vi "io_write.vi"(6 "Block Logging (F)":bool, 8 "error in":errorcluster, 10 "write buffer":string, 11 "VISA resource name":refnum<visa-resource-name>) -> (0 "error out":errorcluster, 3 "VISA resource name out":refnum<visa-resource-name>)   [LabVIEW 2014, in "rszvl_rsidr_core.lvlib"]
uses:
  rszvl_rsidr_core.lvlib
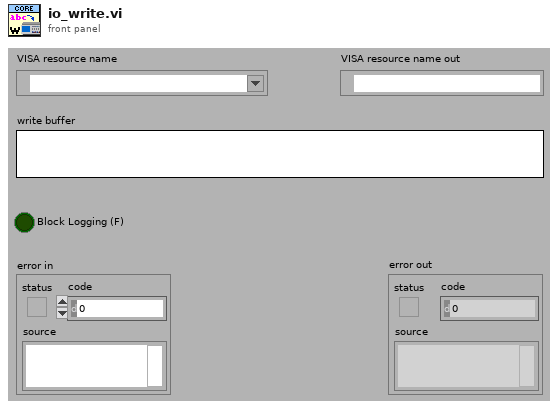
[diagram p1: front panel]
types:
  T1 = typedef "rszvl_rsidr_core.lvlib/type_Session_Data.ctl" = cluster{"Instr type":string, "Instr type for err. msg.":string, "Installed Options":string[], "OPC Timeout":i32, "Query Instrument Status":bool, "Check Range":bool, "Check Options":bool, "Add LF to Write":bool, "Simulate":bool, "Logging":bool, "Logging params":variant, "Interface Type":enum16{"Unknown", "GPIB", "VXI", "GPIB_VXI", "ASRL", "PXI", "TCPIP", "USB", "SOCKET"}, "Fast Sweep":i32, "AdditionalFlags":i32, "WaitBeforeWrite":i32, "WaitBeforeRead":i32, "BinDataChunkSize":i64}
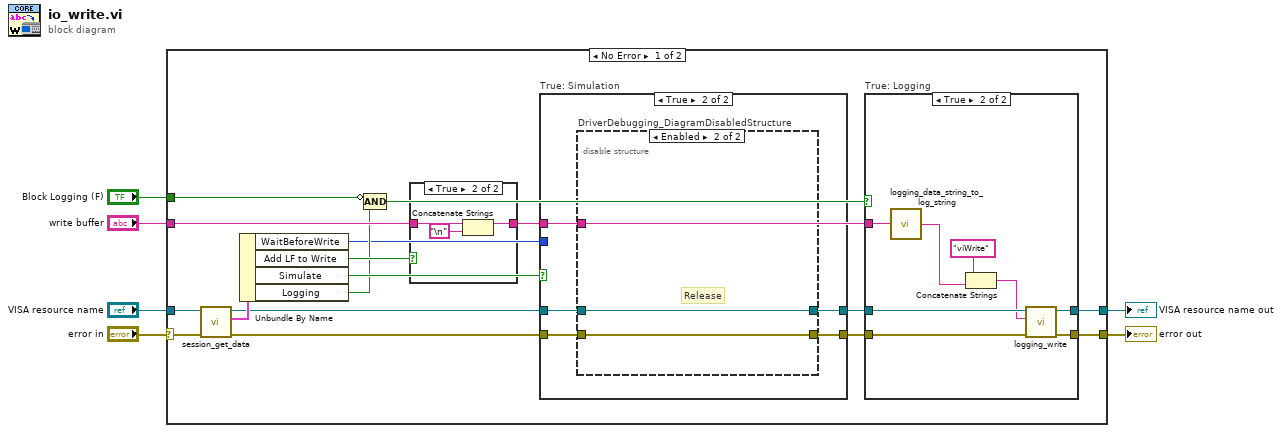
[diagram p0: block diagram]
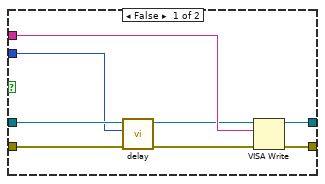
[diagram p3: hidden frame]
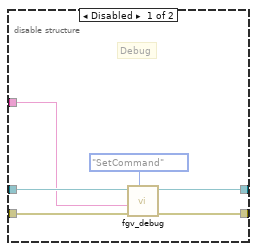
[diagram p4: hidden frame]
diagram:
  n1 = case shown="No Error" "error in" {
    selector: "error in" -> [w20 w60]
    tunnel: [w13 w59] -> w2
    tunnel: [w14 w60] -> w3
    tunnel: "write buffer" -> [w23 _]
    tunnel: "VISA resource name" -> [w19 w59]
    tunnel: "Block Logging (F)" -> [w7 _]
    frame No Error {
      n2 = call "session_get_data.vi"("error in"=w20, "VISA resource name"=w19) -> ("error out"=w18:errorcluster, "Session User Data out"=w21:T1, "VISA resource name out"=w10:refnum<visa-resource-name>)  [unwired: 7 in]
      n3 = Unbundle By Name(w21) -> ("WaitBeforeWrite"=w8:i32, "Add LF to Write"=w22:bool, "Simulate"=w17:bool, "Logging"=w16:bool)
      n4 = Compound Arithmetic op=AND(invert w7, w16) -> (w12:bool)
      n5 = case shown="True" w22 {
        tunnel: w23 -> [w55 w57]
        tunnel: [w55 w58] -> w11
        frame False {
        }
        frame True {
          n6 = Concatenate Strings(w57, "\n" ("Line Feed Constant")) -> (w58:string)
        }
      }
      n7 = case "True: Simulation" shown="True" w17 {
        tunnel: w18 -> [w40 w46]
        tunnel: w10 -> [w39 w45]
        tunnel: [w36 w44] -> w15
        tunnel: w11 -> [w41 w42]
        tunnel: [w35 w43] -> w9
        tunnel: w8 -> [w34 _]
        frame False {
          n8 = call "delay.vi"("error in"=w40, "Milliseconds to wait"=w34, "VISA resource name"=w39) -> ("error out"=w38:errorcluster, "VISA resource name out"=w37:refnum<visa-resource-name>)  [unwired: 7 in]
          n9 = VISA Write(VISA resource name=w37, write buffer=w41, error in (no error)=w38) -> (VISA resource name out=w35:refnum<visa-resource-name>, error out=w36:errorcluster)  [unwired: 1 out]
        }
        frame True {
          n10 = disable-structure "DriverDebugging_DiagramDisabledStructure" shown="Enabled" {
            disable-tunnel: w46 -> [w51 w53]
            disable-tunnel: [w49 w53] -> w44
            disable-tunnel: w45 -> [w50 w54]
            disable-tunnel: [w48 w54] -> w43
            disable-tunnel: w42 -> [w47 _]
            frame Disabled {
              # "Debug"
              n11 = call "fgv_debug.vi"("Operation"=enum16{"Reset", "ReadCommand", "SetCommand"}."SetCommand", "error in"=w51, "Command in"=w47, "VISA resource name"=w50) -> ("error out"=w49:errorcluster, "VISA resource name out"=w48:refnum<visa-resource-name>)  [unwired: 6 in]
            }
            frame Enabled {
              # "Release"
            }
          }
        }
      }
      n12 = case "True: Logging" shown="True" w12 {
        tunnel: [w25 w30] -> w14
        tunnel: [w24 w29] -> w13
        tunnel: w15 -> [w25 w32]
        tunnel: w9 -> [w24 w31]
        tunnel: w11 -> [_ w33]
        frame False {
        }
        frame True {
          n13 = call "logging_data_string_to_log_string.vi"("Raw string to log"=w33) -> ("Result log string"=w28:string)  [unwired: 4 in]
          n14 = Concatenate Strings("viWrite" ("format string"), w28) -> (w26:string)
          n15 = call "logging_write.vi"("error in"=w32, "String to write"=w26, "VISA resource name"=w31) -> ("error out"=w30:errorcluster, "VISA resource name out"=w29:refnum<visa-resource-name>)  [unwired: 7 in]
        }
      }
    }
    frame Error {
    }
  }
  "VISA resource name out" <- w2
  "error out" <- w3
